vi "Core_Get HSMS State.vi"(8 "error in (no error)":errorcluster, 11 "HSMS Class in":refnum<class "HSMS Class.lvclass">) -> (0 "error out":errorcluster, 2 "HSMS State":T1, 3 "HSMS Class out":refnum<class "HSMS Class.lvclass">)   [LabVIEW 2020, in "SECS Communication.lvlib" / "HSMS Class.lvclass"]
uses:
  HSMS Class.lvclass
  HSMS State.ctl
  HSMS Class.lvclass/HSMS Class.ctl
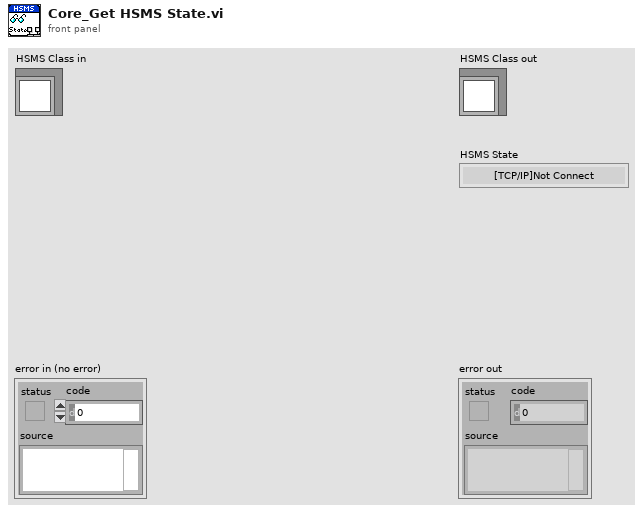
[diagram p1: front panel]
types:
  T1 = typedef "SECS Communication.lvlib/HSMS Class.lvclass/HSMS State.ctl" = enum16{"[TCP/IP]Not Connect", "[HSMS]Not Selected", "[HSMS]Selected", "Stop"}
  T2 = typedef "SECS Communication.lvlib/HSMS Class.lvclass/HSMS State Data.ctl" = cluster{"HSMS State":T1, "T3(Reply Timeout)":i32, "T5(Separation Timeout)":i32, "T6(Control Timeout)":i32, "T7(Not Selected Timeout)":i32, "T8(Inter-Character Timeout)":i32, "Session ID":u16, "Alive Notifier":refnum<notifier>, "Log Path":path, "Listener Refnum":refnum<k5>}
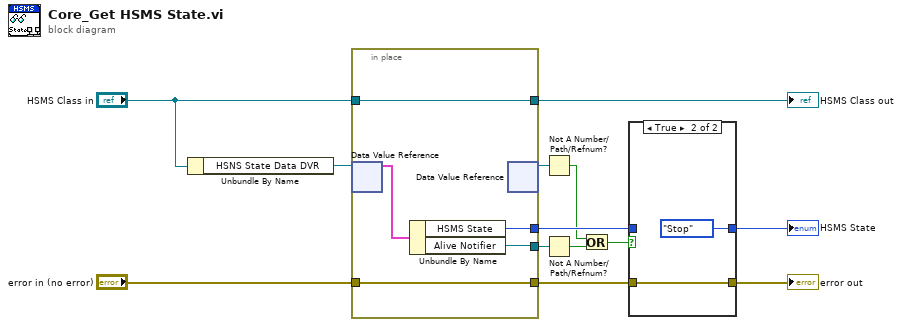
[diagram p0: block diagram]
diagram:
  n1 = Unbundle By Name("HSMS Class in") -> ("HSNS State Data DVR"=w10:refnum<data-value>)
  n2 = in-place {
    in-place-border: "HSMS Class in" -> [w18]
    in-place-border: [w18] -> w12
    in-place-border: [w16] -> w8
    in-place-border: "error in (no error)" -> [w15]
    in-place-border: [w15] -> w6
    in-place-border: [w14] -> w4
    n3 = in-place-dvr #1(w10) -> (w17:T2)  [unwired: 1 out]
    n4 = Unbundle By Name(w17) -> ("HSMS State"=w16:T1, "Alive Notifier"=w14:refnum<notifier>)
    n5 = in-place-dvr #1() -> (w9:refnum<data-value>)  [unwired: 1 in, 1 out]
  }
  "HSMS Class out" <- w12
  n6 = Not A Number/Path/Refnum?(number/path/refnum=w9) -> (NaN/Path/Refnum?=w2:bool)
  n7 = Not A Number/Path/Refnum?(number/path/refnum=w4) -> (NaN/Path/Refnum?=w3:bool)
  n8 = Or(x=w2, y=w3) -> (x .or. y?=w1:bool)
  n9 = case shown="True" w1 {
    tunnel: w8 -> [w20 _]
    tunnel: [w20 HSMS_State."Stop" ("HSMS State")] -> w11
    tunnel: w6 -> [w19 w21]
    tunnel: [w19 w21] -> w5
    frame False {
    }
    frame True {
    }
  }
  "error out" <- w5
  "HSMS State" <- w11
